vi "Tiff Saving module.vi"(0 "data in":sgl[][](array[numeric]), 1 "action":T2=enum."Uninit: close file", 2 "File Type":T1, 7 "Convert to U16?":bool, 9 "file path and name":path, 11 "error in (no error)":errorcluster, 12 "# A-lines to save":i32=2048, 13 "#Z pixels to save":i32=100, 14 "ImageDescription":string) -> (6 "save successful?":bool, 15 "error out":errorcluster)   [LabVIEW 2018]
uses:
  Controls/data manager action.ctl
  type defines/file type.ctl
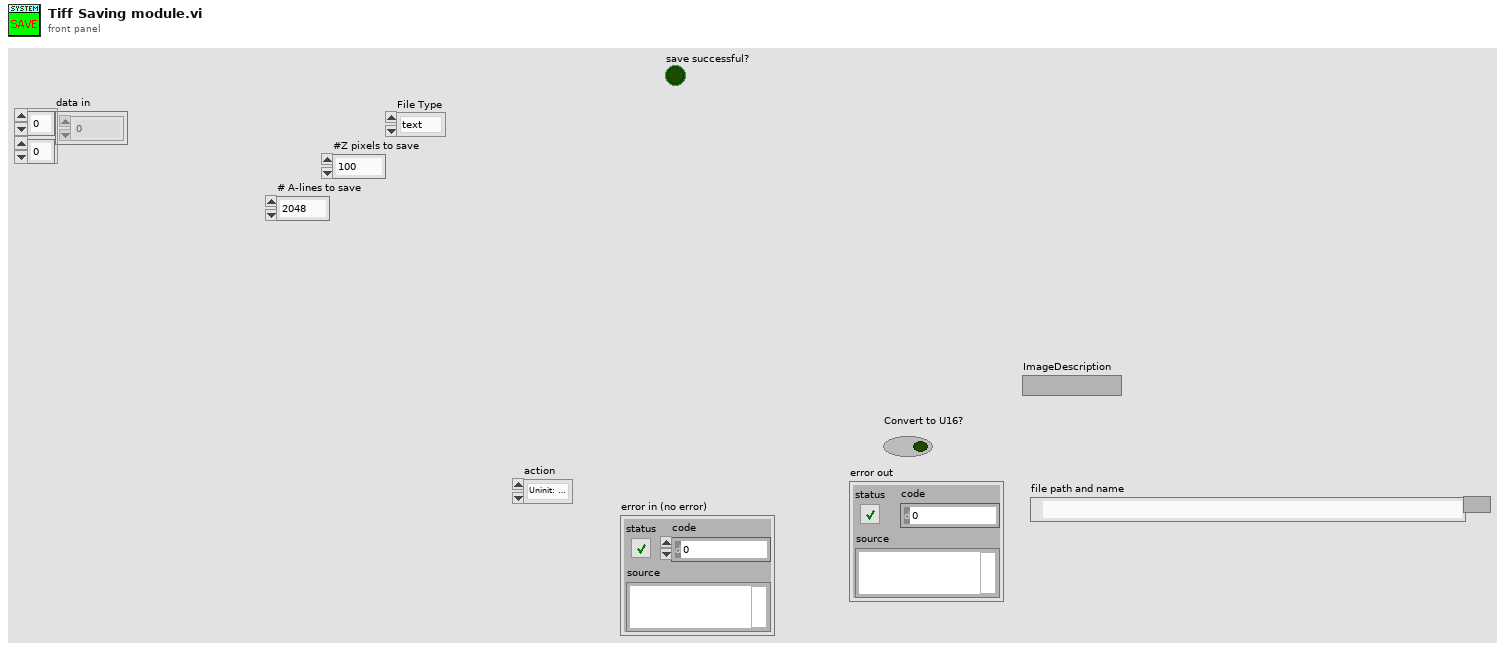
[diagram p1: front panel]
types:
  T1 = typedef "file type.ctl" = enum16{"text", "Tiff", "binary"}
  T2 = typedef "data manager action.ctl" = enum16{"Init: open file", "save", "save as text", "Uninit: close file"}
  T3 = enum16{"open", "replace", "create", "open or create", "replace or create", "replace or create with confirmation"}
  T4 = enum16{"big-endian, network order", "native, host order", "little-endian"}
  T5 = typedef "Image Type" = u32
  T6 = typedef "IMAQ Image.ctl" = refnum<image>
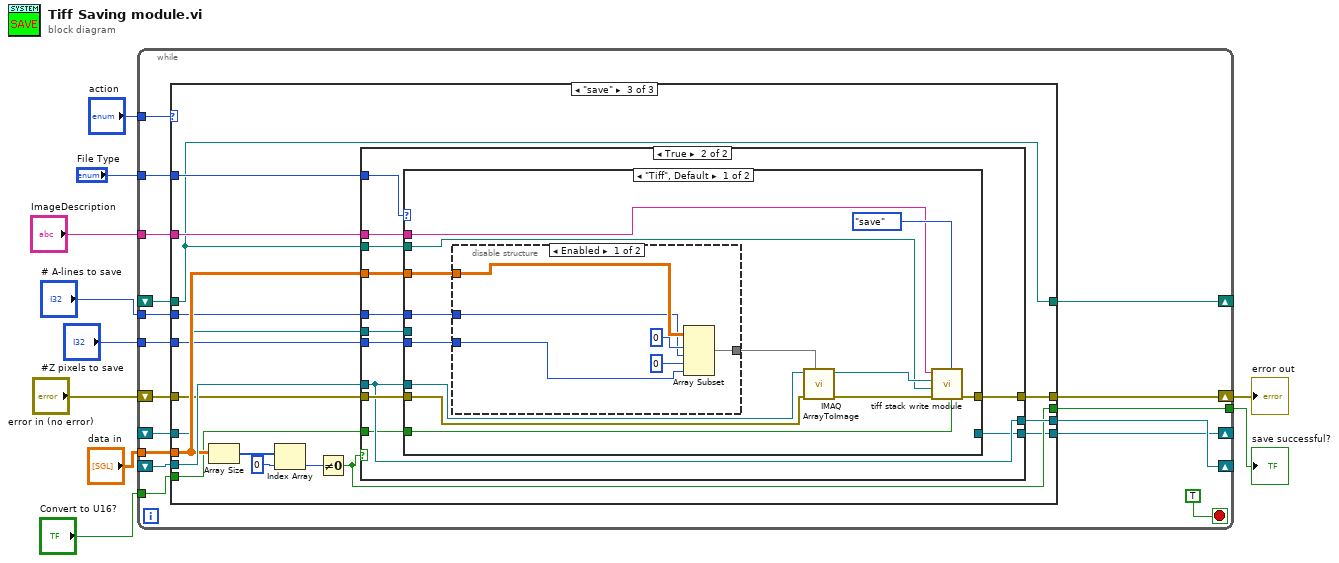
[diagram p0: block diagram]
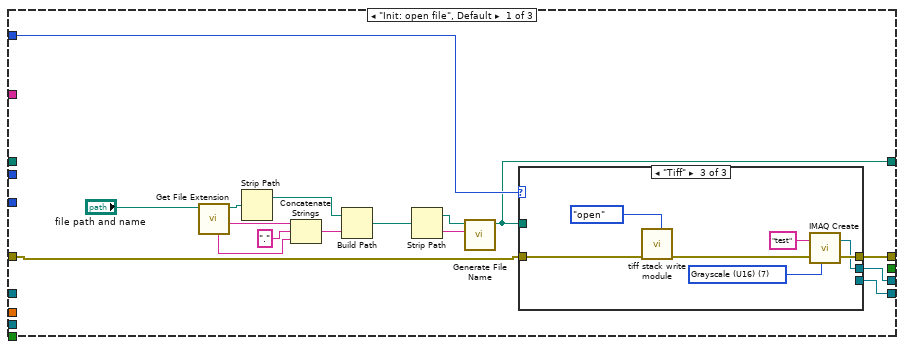
[diagram p2: hidden frame]
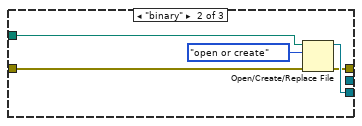
[diagram p4: hidden frame]
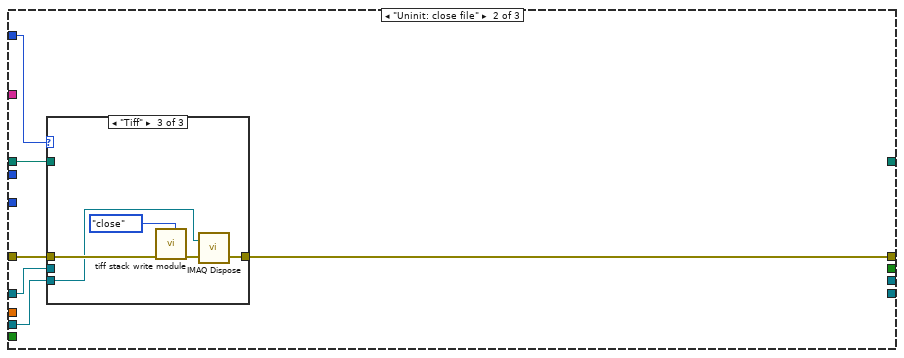
[diagram p5: hidden frame]
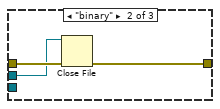
[diagram p7: hidden frame]
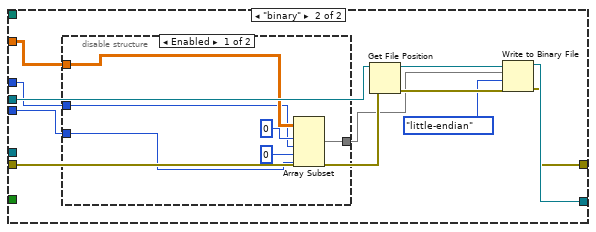
[diagram p10: hidden frame]
diagram:
  n1 = while {
    tunnel: "action" -> [w22]
    shift-right: [w26] -> w9
    shift-left: "error in (no error)" -> [w25]
    shift-right: [w24] -> _
    shift-left: _ -> [w23]
    tunnel: [w21] -> w7
    shift-right: [w20] -> _
    shift-left: _ -> [w19]
    tunnel: "data in" -> [w18]
    tunnel: "Convert to U16?" -> [w17]
    tunnel: "ImageDescription" -> [w16]
    tunnel: "File Type" -> [w15]
    shift-right: [w14] -> _
    shift-left: _ -> [w13]
    tunnel: "# A-lines to save" -> [w12]
    tunnel: "#Z pixels to save" -> [w11]
    stop <- TRUE stop-if-true
    n2 = case shown="\"save\"" w22 {
      tunnel: [w41 w60 w87] -> w26
      tunnel: w25 -> [w43 w62 w83]
      tunnel: [w40 _ w88] -> w24
      tunnel: w23 -> [_ w61 w86]
      tunnel: [_ _ w85] -> w21
      tunnel: [w42 _ w74] -> w20
      tunnel: w19 -> [_ w59 w75]
      tunnel: w18 -> [_ _ w84]
      tunnel: w17 -> [_ _ w82]
      tunnel: w16 -> [_ _ w81]
      tunnel: w15 -> [w29 w58 w80]
      tunnel: [w28 _ w79] -> w14
      tunnel: w13 -> [_ w57 w79]
      tunnel: w12 -> [_ _ w73]
      tunnel: w11 -> [_ _ w72]
      frame "Init: open file", Default {
        n3 = call <vilib>:"Get File Extension.vi"("file"="file path and name") -> ("filename without extension"=w35:string, "dup file"=w39:path, "unmodified file extension"=w31:string)  [unwired: 6 in, 2 out]
        n4 = Strip Path(path=w39) -> (stripped path=w37:path)  [unwired: 1 out]
        n5 = Concatenate Strings(w35, "." ("string"), w31) -> (w38:string)
        n6 = Build Path(base path=w37, name or relative path=w38) -> (appended path=w32:path)
        n7 = Strip Path(path=w32) -> (stripped path=w33:path, name=w34:string)
        n8 = call "Generate File Name.vi"("name or relative path"=w34, "base path"=w33) -> ("appended path"=w28:path)  [unwired: 9 in]
        n9 = case shown="\"Tiff\"" w29 {
          tunnel: w43 -> [w44 w48 w55]
          tunnel: [w44 w46 w51] -> w41
          tunnel: [_ w47 _] -> w42
          tunnel: [_ _ w50] -> w40
          tunnel: w28 -> [_ w45 _]
          frame "text", Default {
          }
          frame "binary" {
            n10 = Open/Create/Replace File(file path (use dialog)=w45, error in=w48, operation (0:open)=T3."open or create") -> (refnum out=w47:refnum<file>, error out=w46:errorcluster)  [unwired: 3 in, 1 out]
          }
          frame "Tiff" {
            w53 = T5 7 items=["Grayscale (U8)", "Grayscale (I16)", "Grayscale (SGL)", "Complex (CSG)", "RGB (U32)", "HSL (U32)", "RGB (U64)", "Grayscale (U16)"] ("Image Type")
            n11 = call "tiff stack write module.vi"("action"=enum16{"open", "save", "close"}."open", "error in"=w55) -> ("error out"=w52:errorcluster)  [unwired: 9 in]
            n12 = call "IMAQ Create"("Image Name"="test", "Image Type"=w53, "error in (no error)"=w52) -> ("New Image"=w50:T6, "error out"=w51:errorcluster)  [unwired: 2 in]
          }
        }
      }
      frame "Uninit: close file" {
        n13 = case shown="\"Tiff\"" w58 {
          tunnel: w62 -> [w63 w66 w70]
          tunnel: w61 -> [_ _ w68]
          tunnel: [w63 w64 w67] -> w60
          tunnel: w59 -> [_ w65 _]
          tunnel: w57 -> [_ _ _]
          frame "text", Default {
          }
          frame "binary" {
            n14 = Close File(refnum=w65, error in=w66) -> (error out=w64:errorcluster)  [unwired: 1 out]
          }
          frame "Tiff" {
            n15 = call "tiff stack write module.vi"("action"=enum16{"open", "save", "close"}."close", "error in"=w70) -> ("error out"=w71:errorcluster)  [unwired: 9 in]
            n16 = call "IMAQ Dispose"("Image"=w68, "error in (no error)"=w71) -> ("error out"=w67:errorcluster)  [unwired: 4 in]
          }
        }
      }
      frame "save" {
        n17 = Array Size(array=w84) -> (size(s)=w78:i32[])
        n18 = Index Array(array=w78, index=0) -> (element=w76:i32)
        n19 = Not Equal To 0?(x=w76) -> (x != 0?=w85:bool)
        n20 = case shown="True" w85 {
          tunnel: w84 -> [_ w95]
          tunnel: [w89 w100] -> w88
          tunnel: [w90 w102] -> w87
          tunnel: w86 -> [w89 w100]
          tunnel: w83 -> [w90 w101]
          tunnel: w82 -> [_ w99]
          tunnel: w81 -> [_ w98]
          tunnel: w80 -> [_ w97]
          tunnel: w79 -> [_ w96]
          tunnel: w75 -> [_ w94]
          tunnel: [_ w93] -> w74
          tunnel: w73 -> [_ w92]
          tunnel: w72 -> [_ w91]
          frame False {
          }
          frame True {
            n21 = case shown="\"Tiff\", Default" w97 {
              tunnel: [w112 w128] -> w102
              tunnel: w100 -> [w115 _]
              tunnel: w95 -> [w107 w126]
              tunnel: w101 -> [w114 w132]
              tunnel: w99 -> [w109 _]
              tunnel: w98 -> [w108 _]
              tunnel: w96 -> [w106 _]
              tunnel: w94 -> [_ w133]
              tunnel: [_ w129] -> w93
              tunnel: w92 -> [w104 w125]
              tunnel: w91 -> [w103 w124]
              frame "Tiff", Default {
                n22 = disable-structure shown="Enabled" {
                  disable-tunnel: w107 -> [w121 w122]
                  disable-tunnel: [w118 _] -> w105
                  disable-tunnel: w104 -> [w117 _]
                  disable-tunnel: w103 -> [w116 _]
                  frame Enabled {
                    n23 = Array Subset(array=w121, index (row)=0 ("index"), length (row)=w117, index (col)=0 ("index"), length (col)=w116) -> (w118:sgl[][])
                  }
                  frame Disabled {
                  }
                }
                n24 = call "IMAQ ArrayToImage"("Image Pixels (U16)"=w105, "error in (no error)"=w114, "Image"=w115) -> ("error out"=w113:errorcluster, "Image Out"=w111:T6)  [unwired: 7 in]
                n25 = call "tiff stack write module.vi"("Convert to U16?"=w109, "action"=enum16{"open", "save", "close"}."save", "error in"=w113, "file Path"=w106, "Image (U8, U16, I16)"=w111, "ImageDescription"=w108) -> ("error out"=w112:errorcluster)  [unwired: 5 in]
              }
              frame "binary" {
                n26 = disable-structure shown="Enabled" {
                  disable-tunnel: w126 -> [w139 w140]
                  disable-tunnel: [w136 _] -> w123
                  disable-tunnel: w125 -> [w135 _]
                  disable-tunnel: w124 -> [w134 _]
                  frame Enabled {
                    n27 = Array Subset(array=w139, index (row)=0 ("index"), length (row)=w135, index (col)=0 ("index"), length (col)=w134) -> (w136:sgl[][])
                  }
                  frame Disabled {
                  }
                }
                n28 = Get File Position(4:w132, 7:w133) -> (0:w131:errorcluster, 3:w130:refnum<file>)  [unwired: 1 out]
                n29 = Write to Binary File(file (use dialog)=w130, data=w123, error in=w131, 9:T4."little-endian" ("byte order (0:big-endian, network order)")) -> (refnum out=w129:refnum<file>, error out=w128:errorcluster)  [unwired: 2 in, 1 out]
              }
            }
          }
        }
      }
    }
  }
  "error out" <- w9
  "save successful?" <- w7
